vi "motor_move_position.vi"(7 "磁铁最低位置":dbl, 8 "错误输入（无错误）":errorcluster, 10 "target position":dbl, 11 "device index":T1) -> (0 "错误输出":errorcluster, 2 "ont?":bool, 3 "position":dbl)   [LabVIEW 2017]
uses:
  device index.ctl
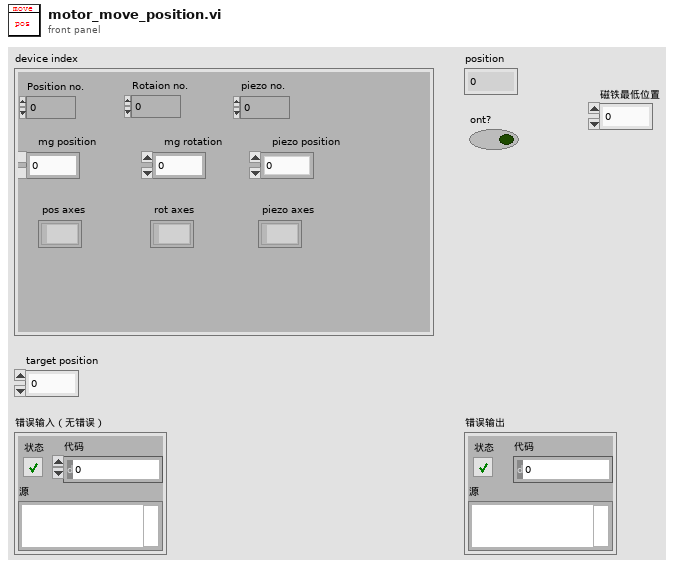
[diagram p1: front panel]
types:
  T1 = typedef "device index.ctl" = cluster{"Position no.":i32, "Rotaion no.":i32, "piezo no.":i32, "mg position":dbl, "mg rotation":dbl, "piezo position":dbl, "pos axes":string[], "rot axes":string[], "piezo axes":string[]}
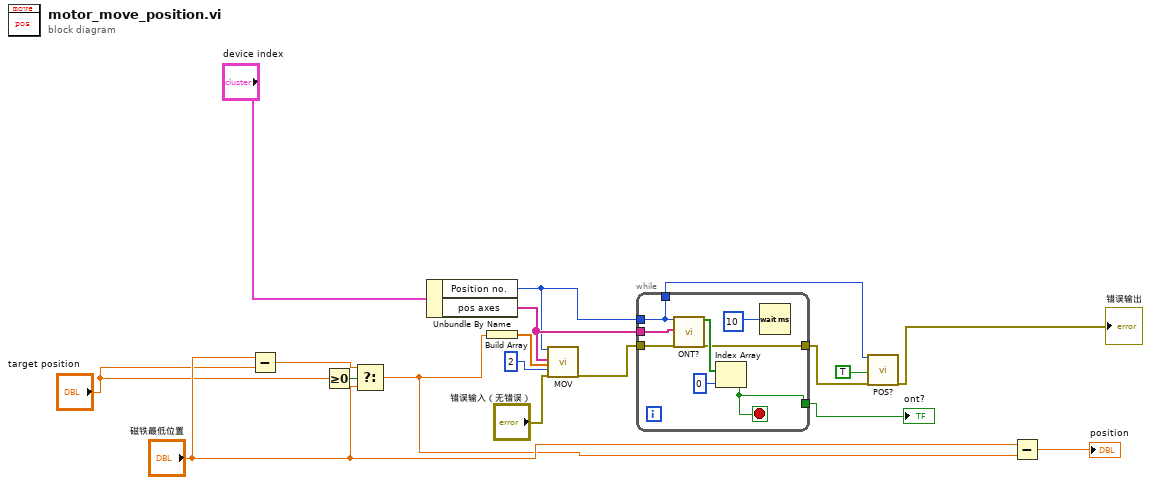
[diagram p0: block diagram]
diagram:
  n1 = Subtract(x="磁铁最低位置", y="target position") -> (x-y=w2:dbl)
  n2 = Greater Or Equal To 0?(x="target position") -> (x >= 0?=w6:bool)
  n3 = Select(t=w2, s=w6, f="磁铁最低位置") -> (s? t:f=w1:dbl)
  n4 = Unbundle By Name("device index") -> ("Position no."=w12:i32, "pos axes"=w13:string[])
  n5 = Build Array(w1) -> (w7:dbl[])
  n6 = call "MOV.vi"("System no."=w12, "Axes to move"=w13, "Position values"=w7, "No.of digits"=i16 2, "error in"="错误输入（无错误）") -> ("error out"=w14:errorcluster)  [unwired: 14 in]
  n7 = while {
    tunnel: w12 -> [w20]
    tunnel: w13 -> [w26]
    tunnel: w14 -> [w25]
    tunnel: [w22] -> w15
    tunnel: [w20] -> w17
    tunnel: [w19] -> w18
    stop <- w19 stop-if-true
    n8 = call "ONT?.vi"("System no."=w20, "Axes to query"=w26, "error in"=w25) -> ("Axis on target?"=w24:bool[], "error out"=w22:errorcluster)  [unwired: 15 in]
    n9 = Index Array(array=w24, index=0 ("索引")) -> (element=w19:bool)
    n10 = Wait (ms)(milliseconds to wait=u32 10 ("等待时间（毫秒）")) -> ()  [unwired: 1 out]
  }
  "ont?" <- w18
  n11 = call "POS?.vi"("System no."=w17, "All axes?"=TRUE, "error in"=w15) -> ("error out"=→"错误输出":errorcluster)  [unwired: 15 in, 1 out]
  n12 = Subtract(x="磁铁最低位置", y=w1) -> (x-y=→"position":dbl)
